vi "unused_getStopMechanism.vi"(8 "error in (no error)":errorcluster, 11 "TaskMock in":refnum<class "TaskMock.lvclass">) -> (0 "error out":errorcluster, 2 "stopMechanism":refnum<class "ITaskStopMechanism.lvclass">, 3 "TaskMock out":refnum<class "TaskMock.lvclass">)   [LabVIEW 2023]
doc: "Returns the stop mechanism type used by the task."
uses:
  TaskMock.lvclass/TaskMock.ctl
  source/BoolNotifierStopMech/BoolNotifierStopMechanism.lvclass
  source/ITaskStopMechanism/ITaskStopMechanism.lvclass
  TaskMock.lvclass
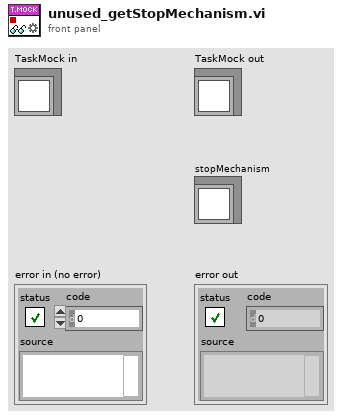
[diagram p1: front panel]
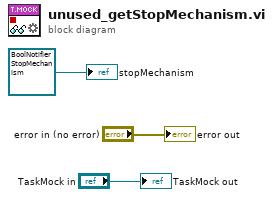
[diagram p0: block diagram]
diagram:
  "error out" <- "error in (no error)"
  "TaskMock out" <- "TaskMock in"
  "stopMechanism" <- refnum<class "BoolNotifierStopMechanism.lvclass"> refnum ("TLC_Daemon.lvlib:NotifierStopMechanism.lvclass")
